vi "Read Msg Output.vi"(10 "Msg Output":refnum<class "Msg Output.lvclass">) -> ()   [LabVIEW 2020, in "jettl.lvlib" / "Stopped jettl Msg.lvlib" / "Stopped Msg Output.lvlib"]
uses:
  Stopped Msg Output.lvlib
  Msg Output/Msg Output.lvclass
  Stopped Msg Output/Stopped Msg Output.lvclass
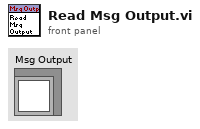
[diagram p1: front panel]
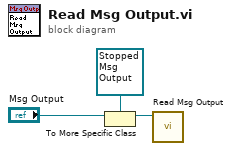
[diagram p0: block diagram]
diagram:
  n1 = To More Specific Class(target class=refnum<class "Stopped Msg Output.lvclass"> refnum ("jettl.lvlib:Stopped jettl Msg.lvlib:Stopped Msg Output.lvlib:Stopped Msg Output.lvclass"), reference="Msg Output") -> (specific class reference=w1:refnum<class "Stopped Msg Output.lvclass">)  [unwired: 1 in, 1 out]
  n2 = call "Read Msg Output.vi"("Stopped Msg Output in"=w1) -> ()  [unwired: 11 in]
